vi "Clear Errors.vi"(8 "error in (no error)":errorcluster, 11 "specific error code to clear (0: all)":i32) -> (0 "error out":errorcluster)   [LabVIEW 2014, in "LVCOOOP.lvlib"]
uses:
  LVCOOOP.lvlib
panel:
  out "specific error cleared?":bool
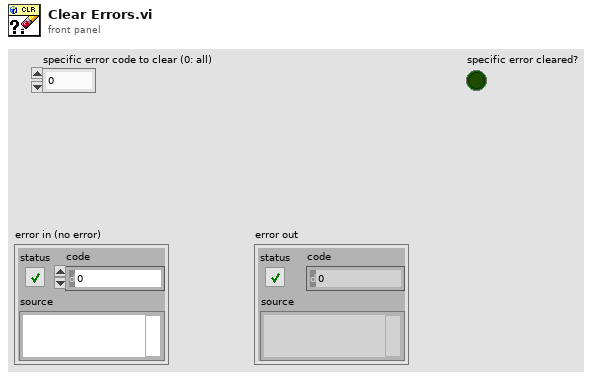
[diagram p1: front panel]
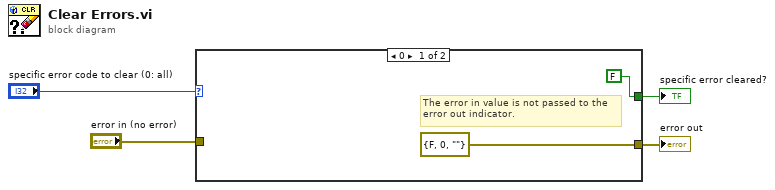
[diagram p0: block diagram]
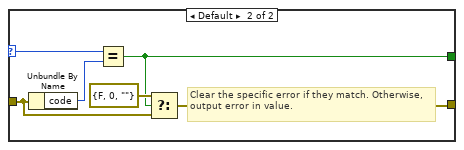
[diagram p2: hidden frame]
diagram:
  n1 = case shown="0" "specific error code to clear (0: all)" {
    selector: "specific error code to clear (0: all)" -> [_ w11]
    tunnel: "error in (no error)" -> [_ w10]
    tunnel: [errorcluster {"status"=FALSE, "code"=0, "source"=""} ("error constant") w7] -> w1
    tunnel: [FALSE w8] -> w3
    frame 0 {
      # "The error in value is not passed to the\nerror out indicator."
    }
    frame Default {
      # "Clear the specific error if they match. Otherwise, output error in value."
      n2 = Unbundle By Name(w10) -> ("code"=w12:i32)
      n3 = Equal?(x=w11, y=w12) -> (x = y?=w8:bool)
      n4 = Select(t=errorcluster {"status"=FALSE, "code"=0, "source"=""} ("error constant"), s=w8, f=w10) -> (s? t:f=w7:errorcluster)
    }
  }
  "error out" <- w1
  "specific error cleared?" <- w3
